vi "Get Channel Block Data References.vi"(8 "error in":errorcluster, 10 "Channel Data Refs":i32[](array[numeric]) format="%.0x") -> (0 "error out":errorcluster, 1 "Values Array":dbl[](array[numeric]), 2 "Block Data Refs":T1(array[cluster]) {"Data Reference" format="%.0x"})   [LabVIEW 2026, in "NIDMM Deployment Hooks.lvlib"]
doc: "Returns an array of 32-bit data references to the inline custom device channels specified by <B>Channel Refs</B>. This VI also returns the channel values. You can use the <B>Block Data Refs</B> with the Get Channel Values by Block Data Reference and Set Channel Values by Block Data Reference VIs."
uses:
  NIDMM Deployment Hooks.lvlib
  <vilib>/NI VeriStand/Custom Device API/Data Reference.ctl
  <vilib>/NI VeriStand/Custom Device API/Custom Device API.lvlib
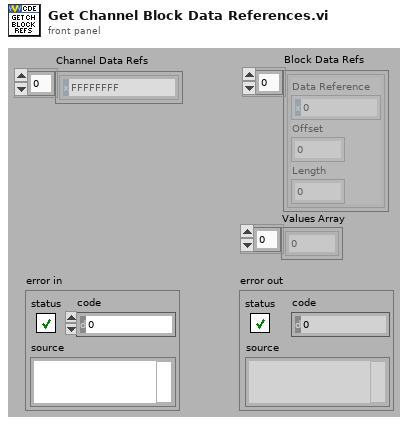
[diagram p1: front panel]
types:
  T1 = cluster{"Data Reference":i32, "Offset":u64, "Length":u64}[]
  T2 = typedef "Custom Device API.lvlib/Data Reference.ctl" = i32
  T3 = cluster{"Data Reference":i32, "Offset":u64, "Length":u64}
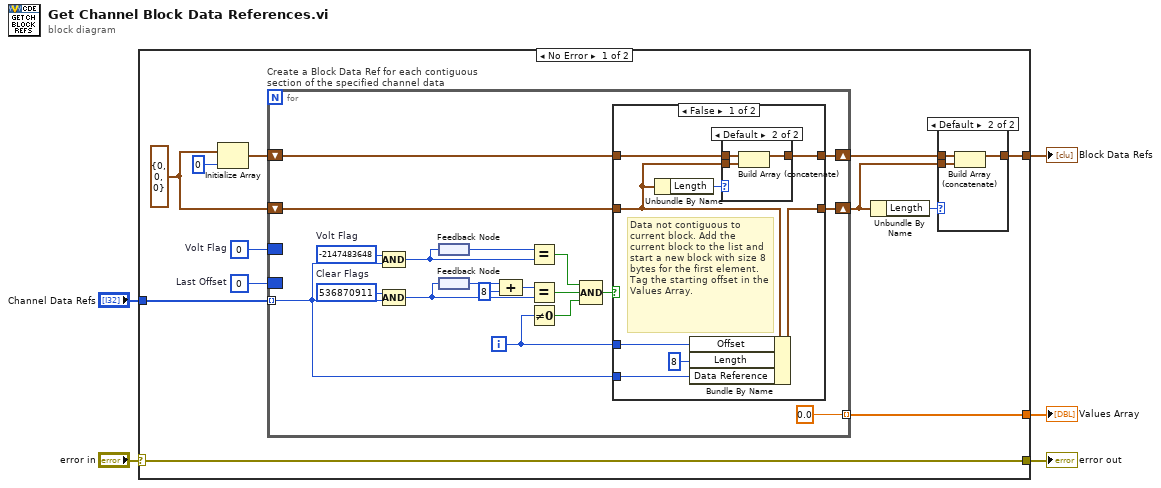
[diagram p0: block diagram]
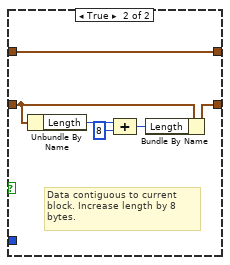
[diagram p4: hidden frame]
diagram:
  n1 = case shown="No Error" "error in" {
    selector: "error in" -> [w6 w59]
    tunnel: [w6 w59] -> w5
    tunnel: "Channel Data Refs" -> [w17 _]
    tunnel: [w12 _] -> w3
    tunnel: [w8 _] -> w1
    frame No Error {
      w14 = T3 {"Data Reference"=0, "Offset"=0, "Length"=0} ("Block Data Ref")
      w9 = 0  # Last Offset
      w10 = 0  # Volt Flag
      n2 = Initialize Array(w14, 0 ("dimension size")) -> (w15:T1)
      n3 = for "Create a Block Data Ref for each contiguous section of the specified channel data" {
        tunnel: w17 -> [w22] mode=indexing
        shift-right: [w30] -> w13
        shift-left: w15 -> [w31]
        border: w9 -> [_]
        shift-right: [w32] -> w11
        shift-left: w14 -> [w40]
        tunnel: [0.0 ("element")] -> w8 mode=indexing
        border: w10 -> [_]
        i -> [w24]
        w38 = 536870911  # Clear Flags
        w39 = -2147483648  # Volt Flag
        n4 = Compound Arithmetic op=AND(w39, w22) -> (w25:i32)
        n5 = Compound Arithmetic op=AND(w38, w22) -> (w35:i32)
        n6 = feedback-in #1(w25) -> ()
        n7 = feedback #1() -> (w26:i32)
        n8 = feedback-in #2(w35) -> ()
        n9 = feedback #2() -> (w36:i32)
        n10 = Compound Arithmetic op=ADD(w36, T2 8 ("value")) -> (w37:T2)
        n11 = Equal?(x=w26, y=w25) -> (x = y?=w28:bool)
        n12 = Equal?(x=w37, y=w35) -> (x = y?=w33:bool)
        n13 = Not Equal To 0?(x=w24) -> (x != 0?=w23:bool)
        n14 = Compound Arithmetic op=AND(w28, w33, w23) -> (w29:bool)
        n15 = case shown="False" w29 {
          tunnel: w40 -> [w45 w58]
          tunnel: [w42 w55] -> w32
          tunnel: w31 -> [w47 w54]
          tunnel: [w46 w54] -> w30
          tunnel: w22 -> [w44 _]
          tunnel: w24 -> [w41 _]
          frame False {
            # "Data not contiguous to current block. Add the current block to the list and start a new block with size 8 bytes for the first element. Tag the starting offset in the Values Array."
            n16 = Unbundle By Name(w45) -> ("Length"=w48:u64)
            n17 = Bundle By Name(cluster=w45, "Offset"=w41, "Length"=u64 8, "Data Reference"=w44) -> (w42:T3)
            n18 = case shown="Default" w48 {
              tunnel: w47 -> [w49 w52]
              tunnel: w45 -> [_ w51]
              tunnel: [w49 w50] -> w46
              frame 0 {
              }
              frame Default {
                n19 = Build Array (concatenate)(w52, w51) -> (w50:T1)
              }
            }
          }
          frame True {
            # "Data contiguous to current block. Increase length by 8 bytes."
            n20 = Unbundle By Name(w58) -> ("Length"=w57:u64)
            n21 = Compound Arithmetic op=ADD(w57, u64 8 ("value")) -> (w56:u64)
            n22 = Bundle By Name(cluster=w58, "Length"=w56) -> (w55:T3)
          }
        }
      }
      n23 = Unbundle By Name(w11) -> ("Length"=w7:u64)
      n24 = case shown="Default" w7 {
        tunnel: w13 -> [w18 w21]
        tunnel: w11 -> [_ w20]
        tunnel: [w18 w19] -> w12
        frame 0 {
        }
        frame Default {
          n25 = Build Array (concatenate)(w21, w20) -> (w19:T1)
        }
      }
    }
    frame Error {
    }
  }
  "error out" <- w5
  "Block Data Refs" <- w3
  "Values Array" <- w1
